vi "LabVIEW Real-Time Serial Initialize.vi"(6 "stop bits (10: 1 bit)":u16(ring)=10 items=["1 bit"=10, "1.5 bits"=15, "2 bits"=20], 7 "Invert Polarity?":bool, 8 "error in (no error)":errorcluster, 9 "parity (0:none)":u16(ring) items=["None", "Odd", "Even", "Mark", "Space"], 10 "data bits (8)":u16=8 min=5 max=8 step=1, 11 "baud rate (9600)":u32=9600) -> (0 "error out":errorcluster, 3 "FPGA VI Reference Out":T1)   [LabVIEW 2012]
doc: "Initializes connection to the serial port."
uses:
  <vilib>/rvi/interface/nirviMethod/nirviMethod.xnode
  <vilib>/rvi/interface/nirviOpenFPGA/nirviOpenFPGA.xnode
  <vilib>/rvi/interface/nirviReadWriteControl/nirviReadWriteControl.xnode
  Program Files (x86)/National Instruments/LabVIEW 2012/examples/robotics/RS-232 with DIO/RS-232 FPGA Main.vi
  Program Files (x86)/National Instruments/LabVIEW 2012/examples/robotics/RS-232 with DIO/FPGA Bitfiles/FPGARS232_FPGATarget_RS-232FPGAMain_GZpp3UKya7w.lvbitx
  <vilib>/FPGAPlugInAG/sbRIO-9631/niLvFpga_Open_sbRIO-9631.vi
  NiFpgaLv.dll
  <vilib>/Utility/error.llb/Error Cluster From Error Code.vi
  <vilib>/rvi/errors/niLvFpgaAdjustHostInterfaceError.vi
  <vilib>/FPGAPlugInAG/sbRIO-9631/niLvFpga_Run_sbRIO-9631.vi
  Program Files (x86)/National Instruments/LabVIEW 2012/examples/robotics/RS-232 with DIO/FPGA Main VI Reference Typedef.ctl
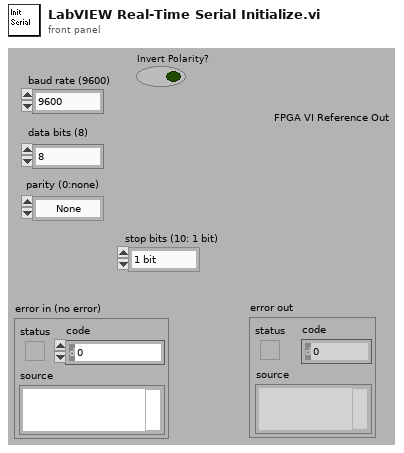
[diagram p1: front panel]
types:
  T1 = typedef "FPGA Main VI Reference Typedef.ctl" = refnum<k20>
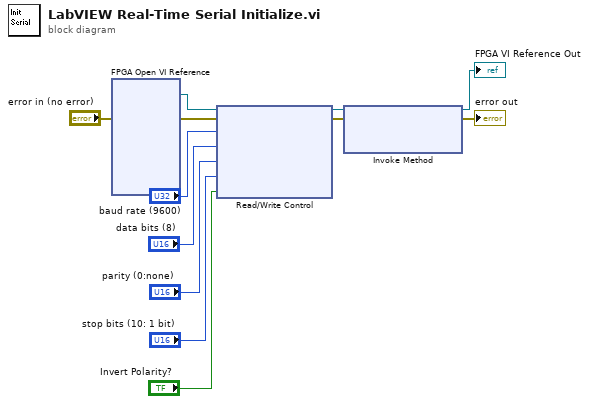
[diagram p0: block diagram]
diagram:
  n1 = xnode "FPGA Open VI Reference"("error in"="error in (no error)") -> ("FPGA VI Reference Out"=w12:refnum<k20>, "error out"=w11:errorcluster)  [unwired: 1 in]
  n2 = xnode "Read/Write Control"("FPGA VI Reference In"=w12, "error in"=w11, "baud rate (9600)"="baud rate (9600)", "data bits (8)"="data bits (8)", "parity (0:none)"="parity (0:none)", "stop bits (10: 1 bit)"="stop bits (10: 1 bit)", "Invert Polarity?"="Invert Polarity?") -> ("FPGA VI Reference Out"=w6:refnum<k20>, "error out"=w5:errorcluster)
  n3 = xnode "Invoke Method"("FPGA VI Reference In"=w6, "error in"=w5) -> ("FPGA VI Reference Out"=→"FPGA VI Reference Out":refnum<k20>, "error out"=→"error out":errorcluster)  [unwired: 1 in]
